vi "DAQmx Write (Digital Bool 1Line 1Point).vi"(0 "task in":refnum<class "Session Factory.lvclass">, 1 "auto start":bool=TRUE, 7 "data":bool, 9 "timeout":dbl=10.0 format="%0.2f", 11 "error in":errorcluster) -> (4 "task out":refnum<class "Session Factory.lvclass">, 10 "number of samples written per channel":u32, 15 "error out":errorcluster)   [LabVIEW 2021, in "Session Management niDAQmx.lvlib" / "Session Factory.lvclass"]
doc: "Writes a single Boolean sample to a task that contains a digital output channel composed of a single line."
uses:
  Session Factory.lvclass
  NI_DAQmx_client/RPC Messages/nidaqmx_grpc_WriteDigitalLinesRequest.ctl
  NI_DAQmx_client/RPC Messages/nidevice_grpc_Session.ctl
  NI_DAQmx_client/RPC Messages/nidevice_grpc_Session_session/nidevice_grpc_Session_session.lvclass
  NI_DAQmx_client/RPC Messages/nidaqmx_grpc_WriteDigitalLinesRequest_data_layout_enum/nidaqmx_grpc_WriteDigitalLinesRequest_data_layout_enum.lvclass
  Session Factory.lvclass/Session Factory.ctl
  NI_DAQmx_client/NI_DAQmx_client.lvlib
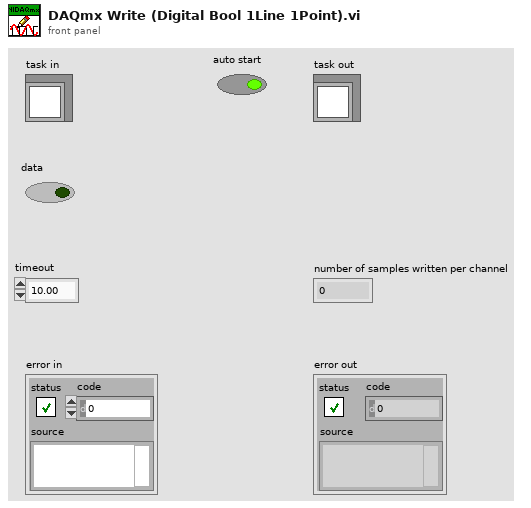
[diagram p1: front panel]
types:
  T1 = typedef "NI_DAQmx_client.lvlib/nidaqmx_grpc_WriteDigitalLinesRequest.ctl" = cluster{"task":T2, "num_samps_per_chan":i32, "auto_start":bool, "timeout":dbl, "nidaqmx_grpc_WriteDigitalLinesRequest_data_layout_enum":refnum<class "nidaqmx_grpc_WriteDigitalLinesRequest_data_layout_enum.lvclass">, "write_array":u8[]}
  T2 = typedef "NI_DAQmx_client.lvlib/nidevice_grpc_Session.ctl" = cluster{"nidevice_grpc_Session_session":refnum<class "nidevice_grpc_Session_session.lvclass">}
  T3 = typedef "grpc-lvsupport-release.lvlib/grpcId.ctl" = u64
  T4 = typedef "NI_DAQmx_client.lvlib/nidaqmx_grpc_WriteDigitalLinesResponse.ctl" = cluster{"status":i32, "samps_per_chan_written":i32}
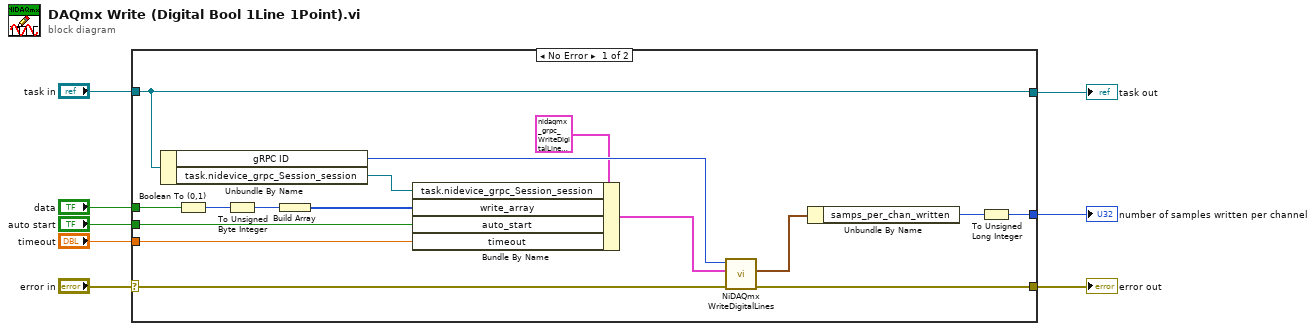
[diagram p0: block diagram]
diagram:
  n1 = case shown="No Error" "error in" {
    selector: "error in" -> [w24 w26]
    tunnel: [w23 w26] -> w7
    tunnel: "task in" -> [w22 w25]
    tunnel: [w22 w25] -> w5
    tunnel: "auto start" -> [w18 _]
    tunnel: "data" -> [w15 _]
    tunnel: "timeout" -> [w16 _]
    tunnel: [w9 _] -> w1
    frame No Error {
      n2 = Unbundle By Name(w22) -> ("gRPC ID"=w21:T3, "task.nidevice_grpc_Session_session"=w19:refnum<class "nidevice_grpc_Session_session.lvclass">)
      n3 = Boolean To (0,1)(Boolean=w15) -> (0, 1=w14:i16)
      n4 = To Unsigned Byte Integer(number=w14) -> (unsigned 8bit integer=w13:u8)
      n5 = Build Array(w13) -> (w12:u8[])
      n6 = Bundle By Name(cluster=T1 {"task"={"nidevice_grpc_Session_session"=refnum}, "num_samps_per_chan"=0, "auto_start"=FALSE, "timeout"=0.0, "nidaqmx_grpc_WriteDigitalLinesRequest_data_layout_enum"=refnum, "write_array"=[]} ("Request Data"), "task.nidevice_grpc_Session_session"=w19, "write_array"=w12, "auto_start"=w18, "timeout"=w16) -> (w17:T1)
      n7 = call "NiDAQmx WriteDigitalLines.vi"("error in"=w24, "Request Data"=w17, "gRPC ID"=w21) -> ("error out"=w23:errorcluster, "Response Data"=w11:T4)  [unwired: 6 in, 1 out]
      n8 = Unbundle By Name(w11) -> ("samps_per_chan_written"=w10:i32)
      n9 = To Unsigned Long Integer(number=w10) -> (unsigned 32bit integer=w9:u32)
    }
    frame Error {
    }
  }
  "error out" <- w7
  "task out" <- w5
  "number of samples written per channel" <- w1
